vi "Test Set Row Values Strings.vi"(11 "Test Case In":refnum<class "Test Open Xml.lvclass">) -> (0 "error out":errorcluster, 3 "Test Case Out":refnum<class "Test Open Xml.lvclass">)   [LabVIEW 2020, in "Test Open Xml.lvclass"]
uses:
  Test Open Xml.lvclass
  <vilib>/Astemes/LUnit/Test Case.lvclass
  Source/Open Xml.lvlib
  Source/Cell DataType.ctl
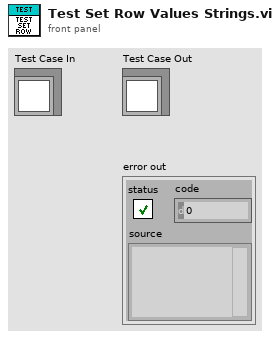
[diagram p1: front panel]
types:
  T1 = typedef "Open Xml.lvlib/Cell DataType.ctl" = enum16{"Void", "Boolean", "Number", "Error", "SharedString", "String", "InlineString", "Date"}
  T2 = cluster{"Number":dbl, "String":string, "Boolean":bool, "Time Stamp":timestamp, "Error":errorcluster}[]
  T3 = cluster{"Number":dbl, "String":string, "Boolean":bool, "Time Stamp":timestamp, "Error":errorcluster}
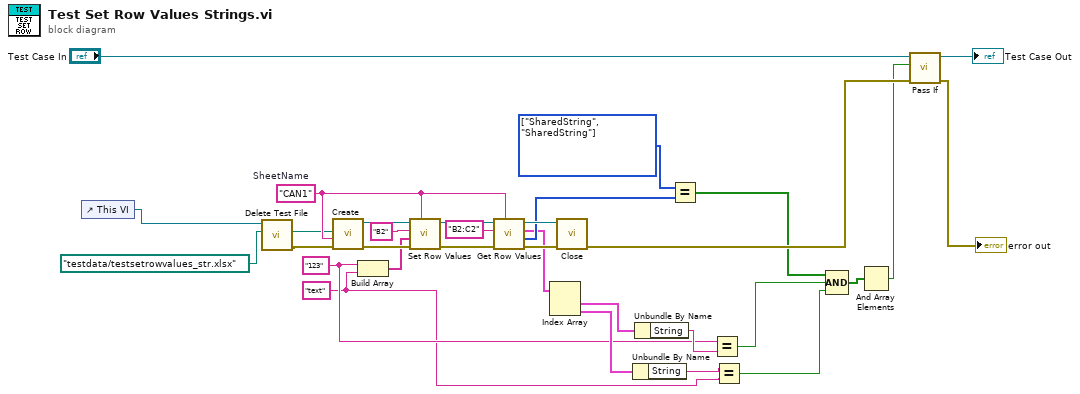
[diagram p0: block diagram]
diagram:
  w15 = T1[] [enum."SharedString", enum."SharedString"] items=["Void", "Boolean", "Number", "Error", "SharedString", "String", "InlineString", "Date"] ("x")
  w6 = "text"
  w10 = "123"
  w24 = "CAN1"  # SheetName
  n1 = control-ref of="This VI"() -> (w1:refnum<vi>)
  n2 = call "Delete Test File.vi"("name or relative path"=path "testdata/testsetrowvalues_str.xlsx", "VI in"=w1) -> ("error out"=w4:errorcluster, "deleted path"=w3:path)  [unwired: 8 in]
  n3 = call "Create.vi"("error in"=w4, "SheetName"=w24, "Path"=w3) -> ("error out"=w28:errorcluster, "SpreadsheetDoc"=w29:refnum<k24>)  [unwired: 7 in]
  n4 = Build Array(w10, w6) -> (w9:string[])
  n5 = call "Set Row Values.vi"("Sheet Name"=w24, "error in"=w28, "Values"=w9, "Cell Address"="B2", "SpreadsheetDoc"=w29) -> ("error out"=w22:errorcluster, "SpreadsheetDoc out"=w21:refnum<k24>)  [unwired: 5 in]
  n6 = call "Get Row Values.vi"("Sheet Name"=w24, "error in"=w22, "Cell Addresses"="B2:C2" ("Cell Address"), "SpreadsheetDoc in"=w21) -> ("error out"=w26:errorcluster, "Types"=w20:T1[], "Cell Values"=w16:T2, "SpreadsheetDoc out"=w25:refnum<k24>)  [unwired: 4 in]
  n7 = Index Array(array=w16) -> (element #1=w14:T3, element #2=w13:T3)  [unwired: 2 in]
  n8 = call "Close.vi"("error in"=w26, "SpreadsheetDoc"=w25) -> ("error out"=w27:errorcluster)  [unwired: 9 in]
  n9 = Unbundle By Name(w13) -> ("String"=w7:string)
  n10 = Unbundle By Name(w14) -> ("String"=w11:string)
  n11 = Equal?(x=w15, y=w20) -> (x = y?=w19:bool[])
  n12 = Equal?(x=w10, y=w11) -> (x = y?=w8:bool)
  n13 = Equal?(x=w7, y=w6) -> (x = y?=w5:bool)
  n14 = Compound Arithmetic op=AND(w19, w8, w5) -> (w12:bool[])
  n15 = And Array Elements(Boolean array=w12) -> (logical AND=w23:bool)
  n16 = call <vilib>:"Pass If.vi"("error in (no error)"=w27, "Pass?"=w23, "LUnit Test Case In"="Test Case In") -> ("error out"=→"error out":errorcluster, "LUnit Test Case Out"=→"Test Case Out":refnum<class "Test Open Xml.lvclass">)  [unwired: 7 in]
